vi "InteractiveDemo.vi"   [LabVIEW 2016]
doc: "This VI demonstrates a very easy, interactive way to execute a measurement with a minimum number of involved VIs."
types:
  T1 = cluster{"Devices":refnum<k24>[], "Signals":refnum<k24>[]}
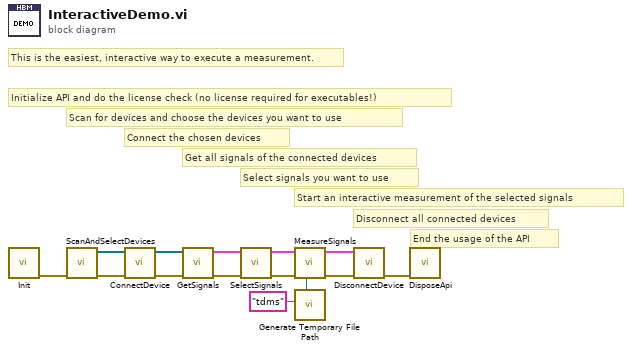
[diagram p0: block diagram]
diagram:
  # "Disconnect all connected devices"
  # "End the usage of the API"
  # "Start an interactive measurement of the selected signals"
  # "This is the easiest, interactive way to execute a measurement."
  # "Select signals you want to use"
  # "Get all signals of the connected devices"
  # "Connect the chosen devices"
  # "Scan for devices and choose the devices you want to use"
  # "Initialize API and do the license check (no license required for executables!)"
  n1 = call "Init.vi"() -> ("Error out"=w8:errorcluster)  [unwired: 8 in, 2 out]
  n2 = call "ScanAndSelectDevices.vi"("Error in"=w8) -> ("Error out"=w14:errorcluster, "SelectedDevices"=w11:refnum<k24>[])  [unwired: 8 in, 1 out]
  n3 = call "ConnectDevice.vi"("Error in"=w14, "Devices"=w11) -> ("Error out"=w13:errorcluster, "Devices"=w10:refnum<k24>[])  [unwired: 7 in, 1 out]
  n4 = call "GetSignals.vi"("Error in"=w13, "Devices"=w10) -> ("Error out"=w12:errorcluster, "DevicesAndSignals"=w9:T1)  [unwired: 7 in, 1 out]
  n5 = call "SelectSignals.vi"("error in (no error)"=w12, "DevicesAndSignals"=w9) -> ("error out"=w7:errorcluster, "DevicesAndSignals"=w6:T1)  [unwired: 7 in, 1 out]
  n6 = call <vilib>:"Generate Temporary File Path.vi"("Temporary File Extension (tmp)"="tdms") -> ("Unique Temporary File Path"=w5:path)  [unwired: 9 in, 1 out]
  n7 = call "MeasureSignals.vi"("Path"=w5, "error in (no error)"=w7, "DevicesAndSignals"=w6) -> ("error out"=w2:errorcluster, "DevicesAndSignals"=w3:T1)  [unwired: 7 in]
  n8 = call "DisconnectDevice.vi"("Error in"=w2, "DevicesAndSignals"=w3) -> ("Error out"=w1:errorcluster)  [unwired: 9 in]
  n9 = call "DisposeApi.vi"("Error in"=w1) -> ()  [unwired: 10 in, 1 out]
